vi "Init Graph Parameters.vi"(8 "error in (no error)":errorcluster, 11 "Top Level in":refnum<class "Top Level.lvclass">) -> (0 "error out":errorcluster, 3 "Top Level out":refnum<class "Top Level.lvclass">)   [LabVIEW 2021, in "Top Level.lvlib" / "Top Level.lvclass"]
uses:
  Top Level.lvclass
  Top Level.lvclass/Top Level.ctl
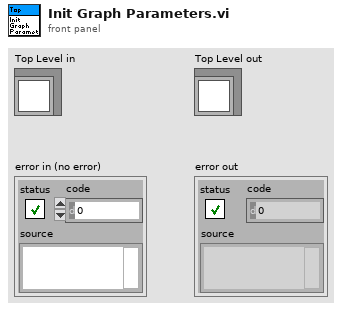
[diagram p1: front panel]
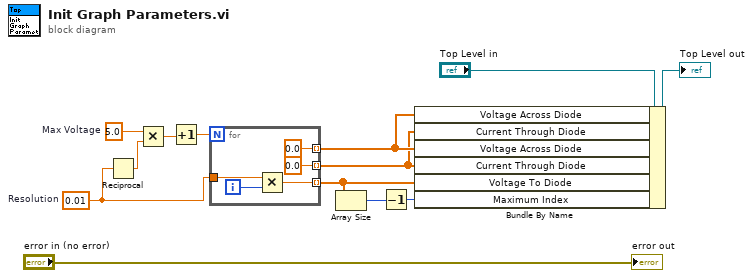
[diagram p0: block diagram]
diagram:
  w9 = 5.0  # Max Voltage
  w8 = 0.01  # Resolution
  n1 = Reciprocal(x=w8) -> (1/x=w10:dbl)
  n2 = Multiply(x=w9, y=w10) -> (x*y=w7:dbl)
  n3 = Increment(x=w7) -> (x+1=w11:dbl)
  n4 = for {
    N: w11 -> [_]
    tunnel: [0.0] -> w1 mode=indexing
    tunnel: w8 -> [w17]
    tunnel: [w15] -> w4 mode=indexing
    tunnel: [0.0] -> w2 mode=indexing
    i -> [w16]
    n5 = Multiply(x=w17, y=w16) -> (x*y=w15:dbl)
  }
  n6 = Array Size(array=w4) -> (size(s)=w6:i32)
  n7 = Decrement(x=w6) -> (x-1=w3:i32)
  n8 = Bundle By Name(cluster="Top Level in", "Voltage Across Diode"=w2, "Current Through Diode"=w1, "Voltage Across Diode"=w2, "Current Through Diode"=w1, "Voltage To Diode"=w4, "Maximum Index"=w3) -> (→"Top Level out":refnum<class "Top Level.lvclass">)
  "error out" <- "error in (no error)"
